vi "Node - Byte Buffer Write.vi"(8 "error in (no error)":errorcluster, 10 "Node Local Channels":T2[](array[typedef]), 11 "Byte Buffer In":refnum<class "Byte Buffer.lvclass">) -> (0 "error out":errorcluster, 1 "Buffer Offsets - Indexes Out":T1[](array[typedef]), 2 "Buffer Offset Out":u64, 3 "Byte Buffer Out":refnum<class "Byte Buffer.lvclass">)   [LabVIEW 2016, in "PXImc Router.lvlib"]
uses:
  PXImc Router.lvlib
  Controls/Node/Node Ch Properties.ctl
  Controls/Data Type.ctl
  <vilib>/NI Veristand/VeriStand Data/Byte Buffer/Byte Buffer.lvclass
  Controls/Node/Node - Buffer Offsets - Indexes.ctl
  <vilib>/NI Veristand/VeriStand Data/Byte Buffer/Byte Buffer.lvclass/Byte Buffer.ctl
  <vilib>/NI Veristand/VeriStand Data/Type Conversion/Type Conversion.From Double (Boolean).vi
  <vilib>/NI Veristand/VeriStand Data/Byte Buffer/Byte Buffer.Write (Boolean).vi
  <vilib>/NI Veristand/VeriStand Data/Type Conversion/Type Conversion.From Double (SGL).vi
  <vilib>/NI Veristand/VeriStand Data/Byte Buffer/Byte Buffer.Write (SGL).vi
  <vilib>/NI Veristand/VeriStand Data/Byte Buffer/Byte Buffer.Write (DBL).vi
  <vilib>/NI Veristand/VeriStand Data/Type Conversion/Type Conversion.From Double (I8).vi
  <vilib>/NI Veristand/VeriStand Data/Byte Buffer/Byte Buffer.Write (I8).vi
  <vilib>/NI Veristand/VeriStand Data/Type Conversion/Type Conversion.From Double (I16).vi
  <vilib>/NI Veristand/VeriStand Data/Byte Buffer/Byte Buffer.Write (I16).vi
  <vilib>/NI Veristand/VeriStand Data/Type Conversion/Type Conversion.From Double (I32).vi
  <vilib>/NI Veristand/VeriStand Data/Byte Buffer/Byte Buffer.Write (I32).vi
  <vilib>/NI Veristand/VeriStand Data/Type Conversion/Type Conversion.From Double (I64).vi
  <vilib>/NI Veristand/VeriStand Data/Byte Buffer/Byte Buffer.Write (I64).vi
  <vilib>/NI Veristand/VeriStand Data/Type Conversion/Type Conversion.From Double (U8).vi
  <vilib>/NI Veristand/VeriStand Data/Byte Buffer/Byte Buffer.Write (U8).vi
  <vilib>/NI Veristand/VeriStand Data/Type Conversion/Type Conversion.From Double (U16).vi
  <vilib>/NI Veristand/VeriStand Data/Byte Buffer/Byte Buffer.Write (U16).vi
  <vilib>/NI Veristand/VeriStand Data/Type Conversion/Type Conversion.From Double (U32).vi
  <vilib>/NI Veristand/VeriStand Data/Byte Buffer/Byte Buffer.Write (U32).vi
  <vilib>/NI Veristand/VeriStand Data/Type Conversion/Type Conversion.From Double (U64).vi
  <vilib>/NI Veristand/VeriStand Data/Byte Buffer/Byte Buffer.Write (U64).vi
  <vilib>/NI Veristand/VeriStand Data/Byte Buffer/Byte Buffer.Write (String).vi
  <vilib>/NI Veristand/VeriStand Data/Byte Buffer/Byte Buffer.Subset.Set.vi
  <vilib>/NI Veristand/VeriStand Data/Byte Buffer/Byte Buffer.Get Buffer Pointer.vi
  <vilib>/NI Veristand/VeriStand Data/Byte Buffer/Byte Buffer.Get Buffer Size.vi
  <vilib>/NI Veristand/VeriStand Data/Memory Management/Memory Management.MoveByteBlock.Read (String).vi
  <vilib>/NI Veristand/VeriStand Data/Byte Buffer/Byte Buffer.Get Byte Order.vi
  <vilib>/NI Veristand/VeriStand Data/Memory Management/Memory Management.Handle Return.vi
  <vilib>/NI Veristand/VeriStand Data/VeriStand Data.lvlib
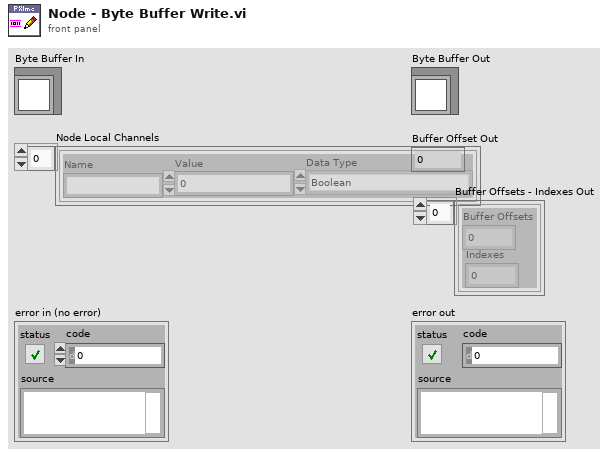
[diagram p1: front panel]
types:
  T1 = typedef "PXImc Router.lvlib/Node - Buffer Offsets - Indexes.ctl" = cluster{"Buffer Offsets":u64, "Indexes":i32}
  T2 = typedef "PXImc Router.lvlib/Node Ch Properties.ctl" = cluster{"Name":string, "Value":dbl, "Data Type":T3}
  T3 = typedef "PXImc Router.lvlib/Data Type.ctl" = enum16{"Boolean", "SGL", "DBL", "I8", "I16", "I32", "I64", "U8", "U16", "U32", "U64"}
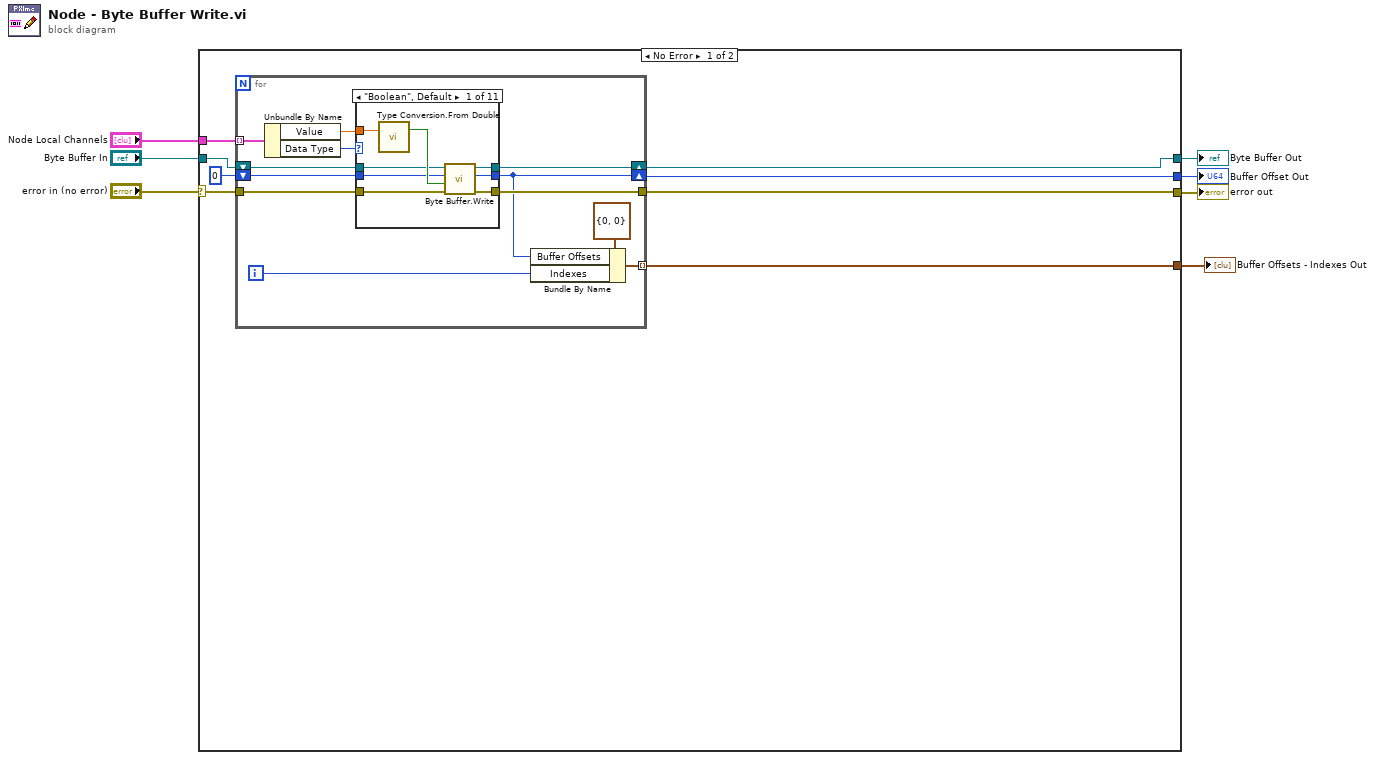
[diagram p0: block diagram]
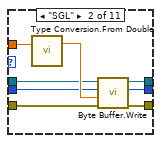
[diagram p2: hidden frame]
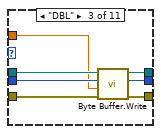
[diagram p3: hidden frame]
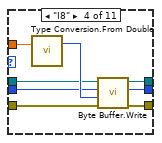
[diagram p4: hidden frame]
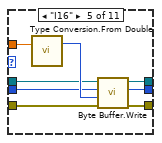
[diagram p5: hidden frame]
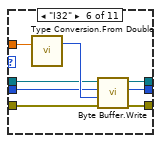
[diagram p6: hidden frame]
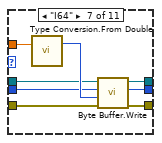
[diagram p7: hidden frame]
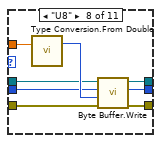
[diagram p8: hidden frame]
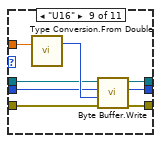
[diagram p9: hidden frame]
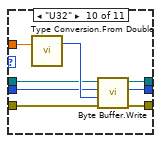
[diagram p10: hidden frame]
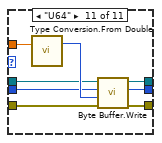
[diagram p11: hidden frame]
diagram:
  n1 = case shown="No Error" "error in (no error)" {
    selector: "error in (no error)" -> [w10 w115]
    tunnel: "Node Local Channels" -> [w15 _]
    tunnel: [w14 _] -> w6
    tunnel: [w8 w115] -> w5
    tunnel: [w13 w116] -> w4
    tunnel: "Byte Buffer In" -> [w11 w116]
    tunnel: [w9 _] -> w1
    frame No Error {
      n2 = for {
        tunnel: [w26] -> w8
        shift-right: [w27] -> w13
        shift-left: w11 -> [w25]
        shift-right: [w19] -> w14
        shift-left: u64 0 ("new buffer offset") -> [w24]
        tunnel: w10 -> [w23]
        tunnel: w15 -> [w22] mode=indexing
        tunnel: [w17] -> w9 mode=indexing
        i -> [w18]
        n3 = Unbundle By Name(w22) -> ("Value"=w16:dbl, "Data Type"=w21:T3)
        n4 = case shown="\"Boolean\", Default" w21 {
          tunnel: [w34 w42 w50 w57 w65 w73 w81 w89 w97 w105 w113] -> w27
          tunnel: [w33 w41 w49 w56 w64 w72 w80 w88 w96 w104 w112] -> w26
          tunnel: w16 -> [w32 w40 w44 w55 w63 w71 w79 w87 w95 w103 w111]
          tunnel: w25 -> [w31 w39 w48 w54 w62 w70 w78 w86 w94 w102 w110]
          tunnel: [w30 w38 w47 w53 w61 w69 w77 w85 w93 w101 w109] -> w19
          tunnel: w24 -> [w28 w37 w46 w52 w60 w68 w76 w84 w92 w100 w108]
          tunnel: w23 -> [w29 w36 w45 w51 w59 w67 w75 w83 w91 w99 w107]
          frame "Boolean", Default {
            n5 = call-poly <vilib>:"Type Conversion.From Double.vi"("value in"=w32) -> ("value out"=w35:bool)  [unwired: 2 in]
            n6 = call-poly <vilib>:"Byte Buffer.Write.vi"("error in (no error)"=w29, "value"=w35, "buffer offset"=w28, "Byte Buffer in"=w31) -> ("error out"=w33:errorcluster, "new buffer offset"=w30:u64, "Byte Buffer out"=w34:refnum<class "Byte Buffer.lvclass">)  [unwired: 5 in]
          }
          frame "SGL" {
            n7 = call-poly <vilib>:"Type Conversion.From Double.vi"("value in"=w40) -> ("value out"=w43:sgl)  [unwired: 2 in]
            n8 = call-poly <vilib>:"Byte Buffer.Write.vi"("error in (no error)"=w36, "value"=w43, "buffer offset"=w37, "Byte Buffer in"=w39) -> ("error out"=w41:errorcluster, "new buffer offset"=w38:u64, "Byte Buffer out"=w42:refnum<class "Byte Buffer.lvclass">)  [unwired: 5 in]
          }
          frame "DBL" {
            n9 = call-poly <vilib>:"Byte Buffer.Write.vi"("error in (no error)"=w45, "value"=w44, "buffer offset"=w46, "Byte Buffer in"=w48) -> ("error out"=w49:errorcluster, "new buffer offset"=w47:u64, "Byte Buffer out"=w50:refnum<class "Byte Buffer.lvclass">)  [unwired: 5 in]
          }
          frame "I8" {
            n10 = call-poly <vilib>:"Type Conversion.From Double.vi"("value in"=w55) -> ("value out"=w58:i8)  [unwired: 2 in]
            n11 = call-poly <vilib>:"Byte Buffer.Write.vi"("error in (no error)"=w51, "value"=w58, "buffer offset"=w52, "Byte Buffer in"=w54) -> ("error out"=w56:errorcluster, "new buffer offset"=w53:u64, "Byte Buffer out"=w57:refnum<class "Byte Buffer.lvclass">)  [unwired: 5 in]
          }
          frame "I16" {
            n12 = call-poly <vilib>:"Type Conversion.From Double.vi"("value in"=w63) -> ("value out"=w66:i16)  [unwired: 2 in]
            n13 = call-poly <vilib>:"Byte Buffer.Write.vi"("error in (no error)"=w59, "value"=w66, "buffer offset"=w60, "Byte Buffer in"=w62) -> ("error out"=w64:errorcluster, "new buffer offset"=w61:u64, "Byte Buffer out"=w65:refnum<class "Byte Buffer.lvclass">)  [unwired: 5 in]
          }
          frame "I32" {
            n14 = call-poly <vilib>:"Type Conversion.From Double.vi"("value in"=w71) -> ("value out"=w74:i32)  [unwired: 2 in]
            n15 = call-poly <vilib>:"Byte Buffer.Write.vi"("error in (no error)"=w67, "value"=w74, "buffer offset"=w68, "Byte Buffer in"=w70) -> ("error out"=w72:errorcluster, "new buffer offset"=w69:u64, "Byte Buffer out"=w73:refnum<class "Byte Buffer.lvclass">)  [unwired: 5 in]
          }
          frame "I64" {
            n16 = call-poly <vilib>:"Type Conversion.From Double.vi"("value in"=w79) -> ("value out"=w82:i64)  [unwired: 2 in]
            n17 = call-poly <vilib>:"Byte Buffer.Write.vi"("error in (no error)"=w75, "value"=w82, "buffer offset"=w76, "Byte Buffer in"=w78) -> ("error out"=w80:errorcluster, "new buffer offset"=w77:u64, "Byte Buffer out"=w81:refnum<class "Byte Buffer.lvclass">)  [unwired: 5 in]
          }
          frame "U8" {
            n18 = call-poly <vilib>:"Type Conversion.From Double.vi"("value in"=w87) -> ("value out"=w90:u8)  [unwired: 2 in]
            n19 = call-poly <vilib>:"Byte Buffer.Write.vi"("error in (no error)"=w83, "value"=w90, "buffer offset"=w84, "Byte Buffer in"=w86) -> ("error out"=w88:errorcluster, "new buffer offset"=w85:u64, "Byte Buffer out"=w89:refnum<class "Byte Buffer.lvclass">)  [unwired: 5 in]
          }
          frame "U16" {
            n20 = call-poly <vilib>:"Type Conversion.From Double.vi"("value in"=w95) -> ("value out"=w98:u16)  [unwired: 2 in]
            n21 = call-poly <vilib>:"Byte Buffer.Write.vi"("error in (no error)"=w91, "value"=w98, "buffer offset"=w92, "Byte Buffer in"=w94) -> ("error out"=w96:errorcluster, "new buffer offset"=w93:u64, "Byte Buffer out"=w97:refnum<class "Byte Buffer.lvclass">)  [unwired: 5 in]
          }
          frame "U32" {
            n22 = call-poly <vilib>:"Type Conversion.From Double.vi"("value in"=w103) -> ("value out"=w106:u32)  [unwired: 2 in]
            n23 = call-poly <vilib>:"Byte Buffer.Write.vi"("error in (no error)"=w99, "value"=w106, "buffer offset"=w100, "Byte Buffer in"=w102) -> ("error out"=w104:errorcluster, "new buffer offset"=w101:u64, "Byte Buffer out"=w105:refnum<class "Byte Buffer.lvclass">)  [unwired: 5 in]
          }
          frame "U64" {
            n24 = call-poly <vilib>:"Type Conversion.From Double.vi"("value in"=w111) -> ("value out"=w114:u64)  [unwired: 2 in]
            n25 = call-poly <vilib>:"Byte Buffer.Write.vi"("error in (no error)"=w107, "value"=w114, "buffer offset"=w108, "Byte Buffer in"=w110) -> ("error out"=w112:errorcluster, "new buffer offset"=w109:u64, "Byte Buffer out"=w113:refnum<class "Byte Buffer.lvclass">)  [unwired: 5 in]
          }
        }
        n26 = Bundle By Name(cluster=T1 {"Buffer Offsets"=0, "Indexes"=0} ("Buffer Offsets - Indexes"), "Buffer Offsets"=w19, "Indexes"=w18) -> (w17:T1)
      }
    }
    frame Error {
    }
  }
  "Buffer Offset Out" <- w6
  "error out" <- w5
  "Byte Buffer Out" <- w4
  "Buffer Offsets - Indexes Out" <- w1
